vi "Initialise.vi"(8 "error in (no error)":errorcluster, 11 "OpenSSL Server Context in":refnum<class "SSL Server Context.lvclass">) -> (0 "error out":errorcluster, 3 "OpenSSL Server Context out":refnum<class "SSL Server Context.lvclass">)   [LabVIEW 2013, in "OpenSSL Socket.lvlib" / "SSL Server Context.lvclass"]
uses:
  SSL Server Context.lvclass
  SSL Context/SSL Context.lvclass/SSL Context.ctl
  SSL Server Context.lvclass/SSL Server Context.ctl
  SSL Context/Read SSL Context.vi
  Read Certificate Chain File.vi
  Read Private Key.vi
  SSL_Lib/SSL-Context/SSL-Context.lvclass
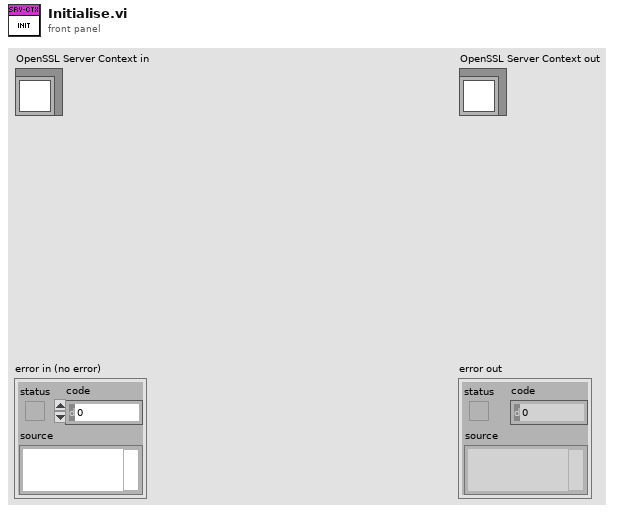
[diagram p1: front panel]
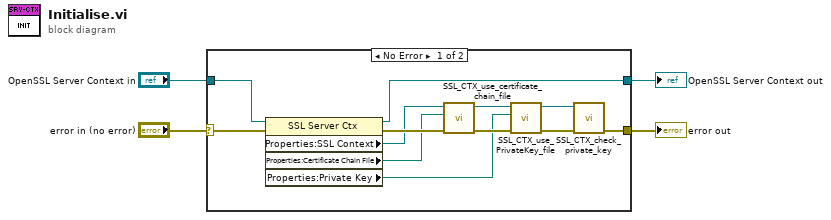
[diagram p0: block diagram]
diagram:
  n1 = case shown="No Error" "error in (no error)" {
    selector: "error in (no error)" -> [w5 w17]
    tunnel: "OpenSSL Server Context in" -> [w16 w18]
    tunnel: [w7 w17] -> w3
    tunnel: [w6 w18] -> w2
    frame No Error {
      n2 = property class="SSL Server Ctx"(reference=w16, error in=w5) -> (reference out=w6:refnum<class "SSL Server Context.lvclass">, error out=w14:errorcluster, "Properties:SSL Context"=w12:refnum<class "SSL-Context.lvclass">, "Properties:Certificate Chain File"=w9:path, "Properties:Private Key"=w8:path)
      n3 = call "SSL_CTX_use_certificate_chain_file.vi"("error in (no error)"=w14, "Certificate Chain File"=w9, "SSL-Context in"=w12) -> ("error out"=w15:errorcluster, "SSL-Context out"=w11:refnum<class "SSL-Context.lvclass">)  [unwired: 7 in]
      n4 = call "SSL_CTX_use_PrivateKey_file.vi"("error in (no error)"=w15, "PrivateKey File"=w8, "SSL-Context in"=w11) -> ("error out"=w13:errorcluster, "SSL-Context out"=w10:refnum<class "SSL-Context.lvclass">)  [unwired: 7 in]
      n5 = call "SSL_CTX_check_private_key.vi"("error in (no error)"=w13, "SSL-Context in"=w10) -> ("error out"=w7:errorcluster)  [unwired: 8 in, 1 out]
    }
    frame Error {
    }
  }
  "error out" <- w3
  "OpenSSL Server Context out" <- w2
